vi "_Caller.vi"() -> ()   [LabVIEW 2019, in "lv-providershell-example1.lvlib"]
uses:
  lv-providershell-example1.lvlib
  src/VIProviderShellHelper.lvclass
panel:
  out "result":dbl=4.0
  in  "a":dbl=4.0
  in  "b":dbl=2.0
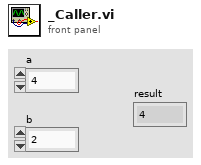
[diagram p1: front panel]
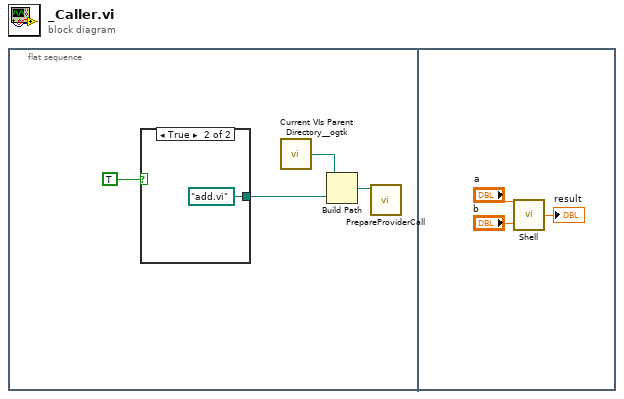
[diagram p0: block diagram]
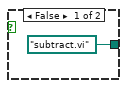
[diagram p2: hidden frame]
diagram:
  n1 = flat-sequence {
    frame #0 {
      n2 = case shown="True" TRUE {
        tunnel: [path "subtract.vi" ("vi path") path "add.vi" ("vi path")] -> w3
        frame False {
        }
        frame True {
        }
      }
      n3 = call <userlib>:"Current VIs Parent Directory__ogtk.vi"() -> ("Parent Directory (+ Relative)"=w4:path)  [unwired: 5 in]
      n4 = Build Path(base path=w4, name or relative path=w3) -> (appended path=w1:path)
      n5 = call "PrepareProviderCall.vi"("ProviderCotentVI Path"=w1) -> ()  [unwired: 10 in, 1 out]
    }
    frame #1 {
      n6 = call "Shell.vi"("b"="b", "a"="a") -> ("result"=→"result":dbl)
    }
  }
